vi "GetTrigTmstmp.vi"(8 "error in (no error)":errorcluster, 10 "TriggerName":T1={"TriggerName"="", "Timeout (s)"=1.0}, 11 "PXI_MultiTrig in":refnum<class "NiPxi6683H.lvclass">) -> (0 "error out":errorcluster, 2 "Timestamp":dbl format="%_6f", 3 "PXI_MultiTrig out":refnum<class "NiPxi6683H.lvclass">)   [LabVIEW 2014, in "SyncPlugins.lvlib" / "NiPxi6683H.lvclass"]
uses:
  NiPxi6683H.lvclass
  SyncPluginBase/Typedefs/clGetTrigTmstmp.ctl
  NiPxi6683H.lvclass/NiPxi6683H.ctl
  SyncPluginBase/SyncPluginBase.lvclass/SyncPluginBase.ctl
  NiPxi6682/NiPxi6682.lvclass/NiPxi6682.ctl
  SyncPluginBase/Accessors/Read PPSTime.vi
  NiPxi6682/Accessors/Read NiSyncHandle.vi
  Accessors/Read Triggers.vi
  <vilib>/Utility/error.llb/Error Cluster From Error Code.vi
  <instrlib>/niSync/niSync.llb/niSync Read Trigger Time Stamp (Single).vi
  <vilib>/ErrorRing/Error Ring.xnode
  SyncPluginBase/SyncPluginBase.lvclass
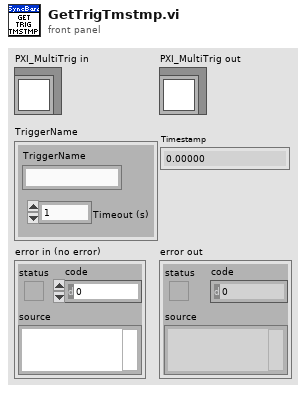
[diagram p1: front panel]
types:
  T1 = typedef "SyncPlugins.lvlib/SyncPluginBase.lvclass/clGetTrigTmstmp.ctl" = cluster{"TriggerName":string, "Timeout (s)":dbl}
  T2 = typedef "SyncPlugins.lvlib/PXI_MultiTrig.lvclass/clTrigger.ctl" = cluster{"Name":string, "DestTerm":string, "SrcTerm":string, "SyncClk":string, "Edge":i32, "Invert?":i32, "Initiated":bool, "Type":string, "TrigTime":bool}
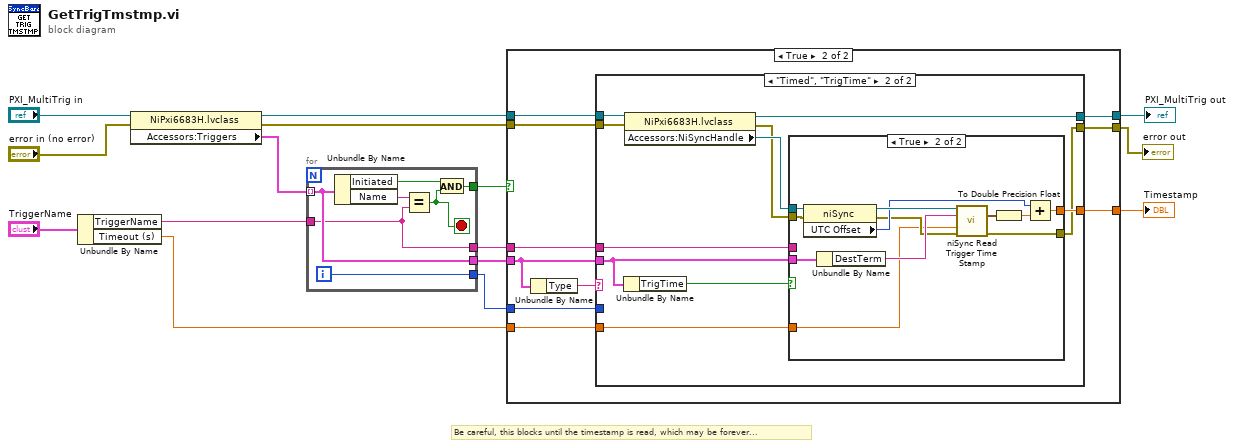
[diagram p0: block diagram]
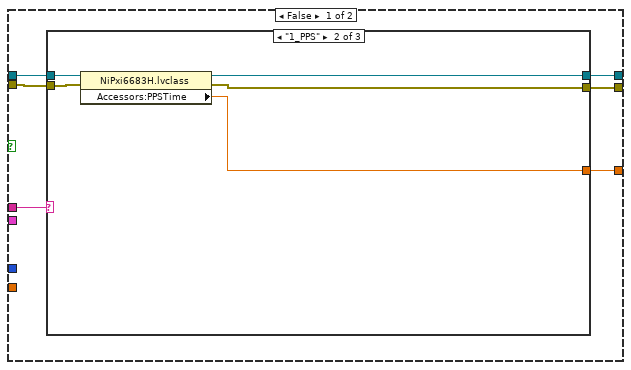
[diagram p2: hidden frame]
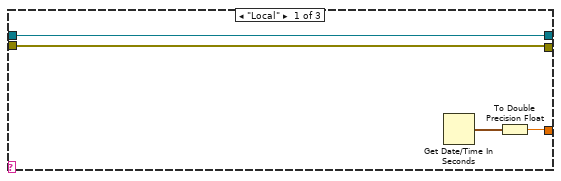
[diagram p3: hidden frame]
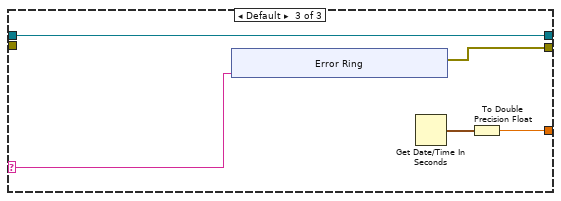
[diagram p4: hidden frame]
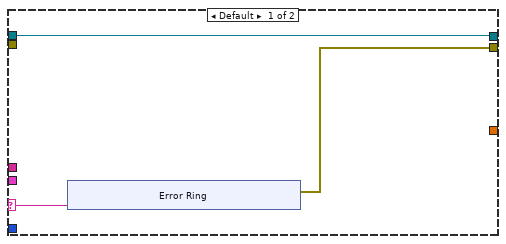
[diagram p5: hidden frame]
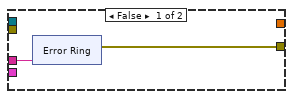
[diagram p6: hidden frame]
diagram:
  # "Be careful, this blocks until the timestamp is read, which may be forever..."
  n1 = Unbundle By Name("TriggerName") -> ("TriggerName"=w2:string, "Timeout (s)"=w1:dbl)
  n2 = property class="NiPxi6683H.lvclass"(reference="PXI_MultiTrig in", error in="error in (no error)") -> (reference out=w10:refnum<class "NiPxi6683H.lvclass">, error out=w6:errorcluster, "Accessors:Triggers"=w12:T2[])
  n3 = for {
    tunnel: w12 -> [w21] mode=indexing
    tunnel: [w21] -> w8
    tunnel: [w18] -> w11
    tunnel: [w17] -> w7
    tunnel: w2 -> [w16]
    tunnel: [w16] -> w9
    i -> [w17]
    stop <- w20 stop-if-true
    n4 = Unbundle By Name(w21) -> ("Initiated"=w19:bool, "Name"=w22:string)
    n5 = Equal?(x=w22, y=w16) -> (x = y?=w20:bool)
    n6 = And(x=w19, y=w20) -> (x .and. y?=w18:bool)
  }
  n7 = case shown="True" w11 {
    tunnel: w10 -> [w26 w54]
    tunnel: w9 -> [w28 w57]
    tunnel: [w25 w51] -> w4
    tunnel: [w27 w58] -> w3
    tunnel: w8 -> [_ w55]
    tunnel: w7 -> [_ w56]
    tunnel: w6 -> [w24 w53]
    tunnel: [w23 w52] -> w5
    tunnel: w1 -> [_ w50]
    frame False {
      n8 = case shown="\"1_PPS\"" w28 {
        selector: w28 -> [_ _ w42]
        tunnel: [w29 w35 w41] -> w27
        tunnel: w26 -> [w30 w37 w40]
        tunnel: [w30 w34 w40] -> w25
        tunnel: w24 -> [w29 w36 _]
        tunnel: [w31 w33 w38] -> w23
        frame "Local" {
          n9 = Get Date/Time In Seconds() -> (seconds since 1Jan1904=w32:timestamp)
          n10 = To Double Precision Float(number=w32) -> (double precision float=w31:dbl)
        }
        frame "1_PPS" {
          n11 = property class="NiPxi6683H.lvclass"(reference=w37, error in=w36) -> (reference out=w34:refnum<class "NiPxi6683H.lvclass">, error out=w35:errorcluster, "Accessors:PPSTime"=w33:dbl)
        }
        frame Default {
          n12 = xnode "Error Ring"("parameter 0"=w42) -> ("error out"=w41:errorcluster)
          n13 = Get Date/Time In Seconds() -> (seconds since 1Jan1904=w39:timestamp)
          n14 = To Double Precision Float(number=w39) -> (double precision float=w38:dbl)
        }
      }
    }
    frame True {
      n15 = Unbundle By Name(w55) -> ("Type"=w59:string)
      n16 = case shown="\"Timed\", \"TrigTime\"" w59 {
        selector: w59 -> [w62 _]
        tunnel: [w61 w71] -> w58
        tunnel: w57 -> [_ w76]
        tunnel: w56 -> [_ _]
        tunnel: w55 -> [_ w75]
        tunnel: w54 -> [w60 w80]
        tunnel: w53 -> [_ w79]
        tunnel: [_ w73] -> w52
        tunnel: [w60 w72] -> w51
        tunnel: w50 -> [_ w70]
        frame Default {
          n17 = xnode "Error Ring"("parameter 0"=w62) -> ("error out"=w61:errorcluster)
        }
        frame "Timed", "TrigTime" {
          n18 = Unbundle By Name(w75) -> ("TrigTime"=w78:bool)
          n19 = property class="NiPxi6683H.lvclass"(reference=w80, error in=w79) -> (reference out=w72:refnum<class "NiPxi6683H.lvclass">, error out=w74:errorcluster, "Accessors:NiSyncHandle"=w77:refnum<k15>)
          n20 = case shown="True" w78 {
            tunnel: w77 -> [_ w100]
            tunnel: w76 -> [w82 _]
            tunnel: w75 -> [_ w101]
            tunnel: w74 -> [_ w97]
            tunnel: [_ w93] -> w73
            tunnel: [w81 w91] -> w71
            tunnel: w70 -> [_ w90]
            frame False {
              n21 = xnode "Error Ring"("parameter 0"=w82) -> ("error out"=w81:errorcluster)
            }
            frame True {
              n22 = property class="niSync"(reference=w100, error in=w97) -> (reference out=w98:refnum<k15>, error out=w92:errorcluster, "UTC Offset"=w94:i32)
              n23 = Unbundle By Name(w101) -> ("DestTerm"=w99:string)
              n24 = call-poly <instrlib>:"niSync Read Trigger Time Stamp.vi"("instrument handle"=w98, "terminal"=w99, "timeout"=w90, "error in (no error)"=w92) -> ("time stamp out"=w96:timestamp, "error out"=w91:errorcluster)  [unwired: 8 in, 2 out]
              n25 = To Double Precision Float(number=w96) -> (double precision float=w95:dbl)
              n26 = Add(x=w94, y=w95) -> (x+y=w93:dbl)
            }
          }
        }
      }
    }
  }
  "error out" <- w3
  "PXI_MultiTrig out" <- w4
  "Timestamp" <- w5
